vi "calculate_ma.vi"(0 "Data_points":i32[](array[numeric]), 5 "Count_size":u64, 11 "error in":errorcluster) -> (4 "Cur_avg":dbl, 15 "error out":errorcluster)   [LabVIEW 2023, in "task-1.lvlib"]
uses:
  <vilib>/Utility/error.llb/DialogType.ctl
  task-1.lvlib
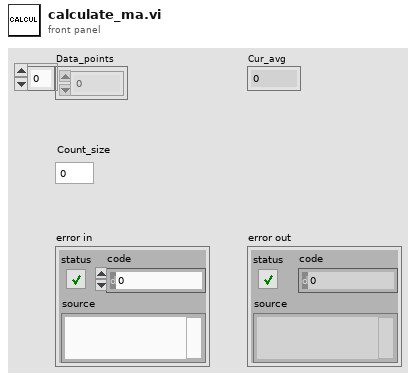
[diagram p1: front panel]
types:
  T1 = typedef "DialogType.ctl" = u16
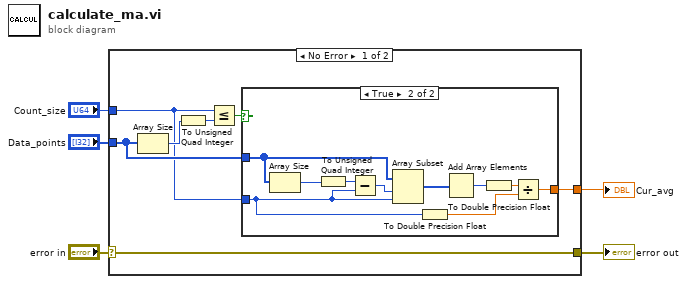
[diagram p0: block diagram]
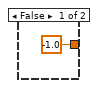
[diagram p2: hidden frame]
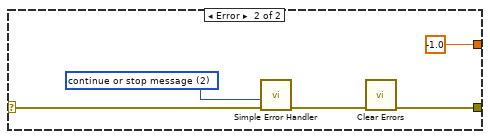
[diagram p3: hidden frame]
diagram:
  n1 = case shown="No Error" "error in" {
    selector: "error in" -> [w12 w28]
    tunnel: [w12 w24] -> w5
    tunnel: "Count_size" -> [w8 _]
    tunnel: "Data_points" -> [w9 _]
    tunnel: [w7 -1.0] -> w3
    frame No Error {
      n2 = Array Size(array=w9) -> (size(s)=w10:i32)
      n3 = To Unsigned Quad Integer(1:w10) -> (0:w6:u64)
      n4 = Less Or Equal?(x=w8, y=w6) -> (x <= y?=w11:bool)
      n5 = case shown="True" w11 {
        tunnel: w9 -> [_ w18]
        tunnel: w8 -> [_ w16]
        tunnel: [-1.0 w19] -> w7
        frame False {
        }
        frame True {
          n6 = Array Size(array=w18) -> (size(s)=w17:i32)
          n7 = To Unsigned Quad Integer(1:w17) -> (0:w14:u64)
          n8 = Subtract(x=w14, y=w16) -> (x-y=w15:u64)
          n9 = Array Subset(array=w18, index=w15, length=w16) -> (w23:i32[])
          n10 = To Double Precision Float(number=w16) -> (double precision float=w21:dbl)
          n11 = Add Array Elements(numeric array=w23) -> (sum=w22:i32)
          n12 = To Double Precision Float(number=w22) -> (double precision float=w20:dbl)
          n13 = Divide(x=w20, y=w21) -> (x/y=w19:dbl)
        }
      }
    }
    frame Error {
      w25 = T1 2 items=["no dialog", "OK message", "continue or stop message", "OK message + warnings", "continue/stop + warnings"] ("type of dialog (OK msg:1)")
      n14 = call <vilib>:"Simple Error Handler.vi"("type of dialog (OK msg:1)"=w25, "error in (no error)"=w28) -> ("error out"=w26:errorcluster)  [unwired: 3 in, 4 out]
      n15 = call <vilib>:"Clear Errors.vi"("error in (no error)"=w26) -> ("error out"=w24:errorcluster)  [unwired: 5 in, 1 out]
    }
  }
  "error out" <- w5
  "Cur_avg" <- w3
